vi "Run.vi"(8 "error in (no error)":errorcluster caption="entrée d'erreur (pas d'erreur)", 9 "X":string[][](array[string]), 10 "Type X":T1(ring), 11 "quantile_transform.lvclass":refnum<class "quantile_transform.lvclass">) -> (0 "error out":errorcluster caption="sortie d'erreur", 2 "Data":T2, 3 "quantile_transform.lvclass":refnum<class "quantile_transform.lvclass">)   [LabVIEW 2020, in "quantile_transform.lvclass"]
doc: "Returns :\n\n- Xt : ndarray or sparse matrix, shape (n_samples, n_features)\nThe transformed data."
uses:
  quantile_transform.lvclass
  quantile_transform.lvclass/quantile_transform.ctl
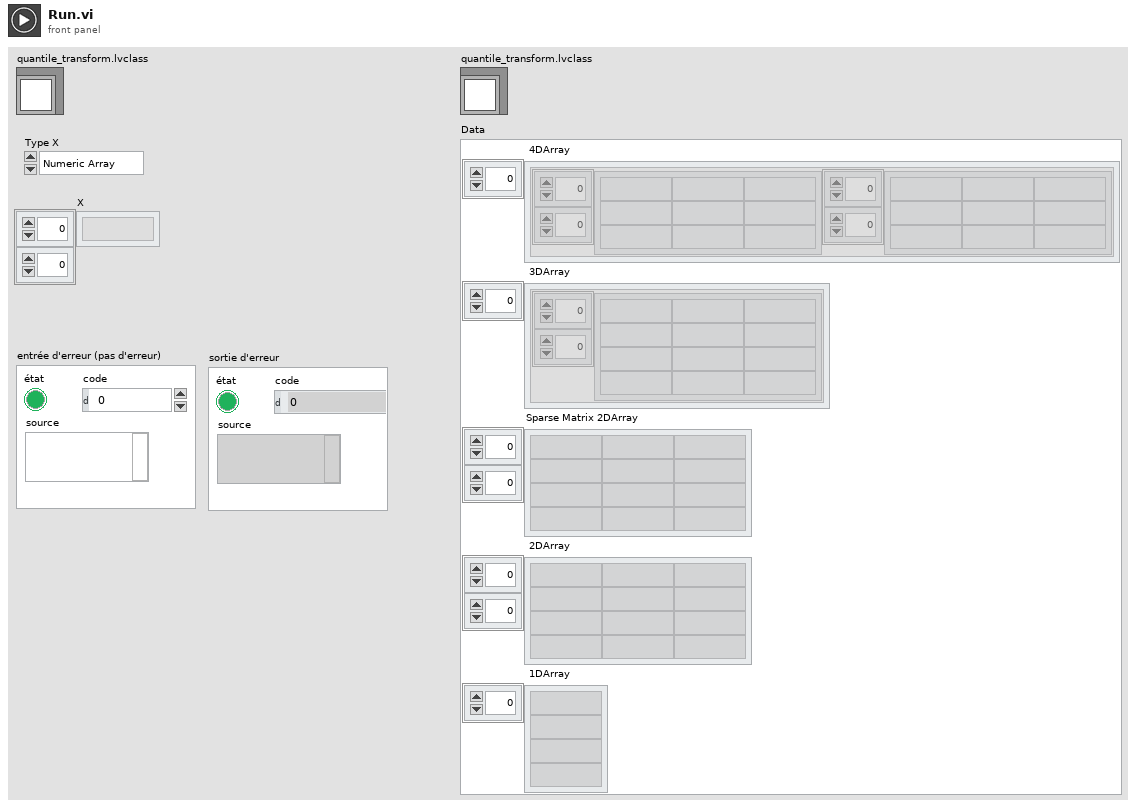
[diagram p1: front panel]
types:
  T1 = enum16{"Numeric Array", "String Array", "Sparse"}
  T2 = cluster{" 4DArray":cluster{"1":string[][], "2":string[][]}[], " 3DArray":cluster{"Tableau":string[][]}[], "Sparse Matrix 2DArray":string[][], " 2DArray":string[][], " 1DArray":string[]}
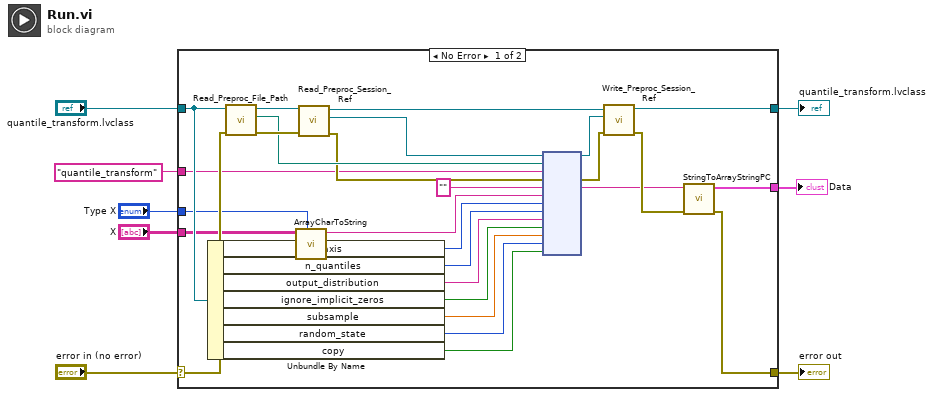
[diagram p0: block diagram]
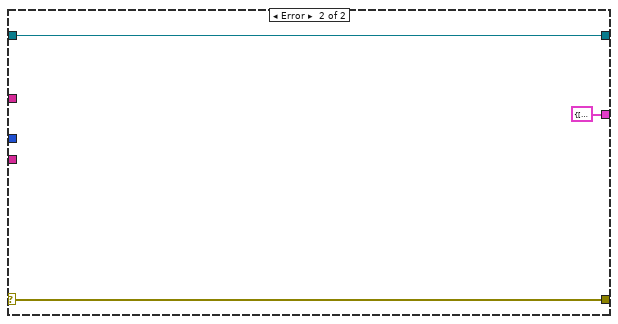
[diagram p2: hidden frame]
diagram:
  n1 = case shown="No Error" "error in (no error)" {
    selector: "error in (no error)" -> [w24 w38]
    tunnel: [w9 w38] -> w7
    tunnel: [w10 w37] -> w5
    tunnel: "quantile_transform.lvclass" -> [w23 w37]
    tunnel: "quantile_transform" ("Fonction") -> [w22 _]
    tunnel: [w11 T2 {" 4DArray"=[], " 3DArray"=[], "Sparse Matrix 2DArray"=[], " 2DArray"=[], " 1DArray"=[]} ("Data")] -> w1
    tunnel: "X" -> [w16 _]
    tunnel: "Type X" -> [w15 _]
    frame No Error {
      n2 = Unbundle By Name(w23) -> ("axis"=w26:i32, "n_quantiles"=w25:i32, "output_distribution"=w21:string, "ignore_implicit_zeros"=w20:bool, "subsample"=w19:dbl, "random_state"=w18:i32, "copy"=w17:bool)
      n3 = call-dynamic "Read_Preproc_File_Path.vi"("error in (no error)"=w24, "Python in"=w23) -> ("error out"=w34:errorcluster, "File_Path"=w31:path, "Python out"=w35:refnum<class "quantile_transform.lvclass">)  [unwired: 7 in]
      n4 = call "ArrayCharToString.vi"("Type"=w15, "TAB"=w16) -> ("Instruction"=w14:string)  [unwired: 9 in]
      n5 = call-dynamic "Read_Preproc_Session_Ref.vi"("error in (no error)"=w34, "Python in"=w35) -> ("error out"=w30:errorcluster, "Session_ref"=w32:refnum<k35>, "Python out"=w33:refnum<class "quantile_transform.lvclass">)  [unwired: 7 in]
      n6 = node(w32, w31, w22, w30, "", w14, w26, w25, w21, w20, w19, w18, w17) -> (w28:refnum<k35>, w29:errorcluster, w12:string)  [unwired: 8 in, 2 out]
      n7 = call-dynamic "Write_Preproc_Session_Ref.vi"("error in (no error)"=w29, "Session_ref"=w28, "Python in"=w33) -> ("error out"=w13:errorcluster, "Python out"=w10:refnum<class "quantile_transform.lvclass">)  [unwired: 7 in]
      n8 = call "StringToArrayStringPC.vi"("sortie d'erreur"=w13, "Return value"=w12) -> ("sortie d'erreur"=w9:errorcluster, "Data"=w11:T2)  [unwired: 8 in]
    }
    frame Error {
    }
  }
  "error out" <- w7
  "quantile_transform.lvclass" <- w5
  "Data" <- w1
